vi "ELVIS III v1.0 Configure DMAs.vi"(7 "DMA Type":string, 8 "error in (no error)":errorcluster, 10 "Channel Names":string[](array[string]), 11 "ELVIS III FPGA Ref":T1) -> (0 "error out":errorcluster, 3 "ELVIS III FPGA Ref":T1)   [LabVIEW 2021]
uses:
  <vilib>/myRIO/Common/Instrument Driver Framework/Utilities/typedefs/Generic FPGA Reference.ctl
  <vilib>/myRIO/Common/Instrument Driver Framework/ELVIS III v1.0/Resource Manager/typedefs/ELVIS III IO Config FPGA Reference.ctl
  <vilib>/myRIO/Common/Instrument Driver Framework/myRIO v1.0/Resource Manager/vis/myRIO v1.0 Block Write Configuration.vi
  <vilib>/rvi/interface/common/niFpgaWaitOnOcc.vi
  <vilib>/rvi/interface/nirviMethod/nirviMethod.xnode
  <vilib>/FPGAPlugInAG/Dynamic/niLvFpga_ConfigureFifo_Dynamic.vi
  <vilib>/rvi/errors/niLvFpgaMergeErrorWithErrorCode.vi
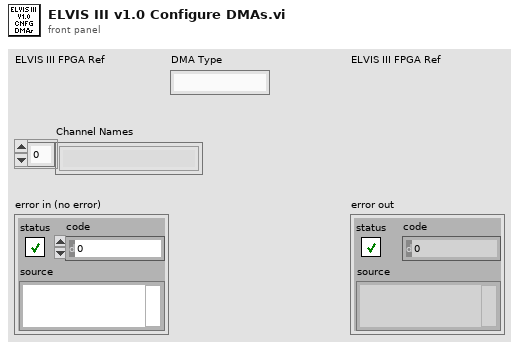
[diagram p1: front panel]
types:
  T1 = typedef "Generic FPGA Reference.ctl" = refnum<k20>
  T2 = typedef "ELVIS III IO Config FPGA Reference.ctl" = refnum<k20>
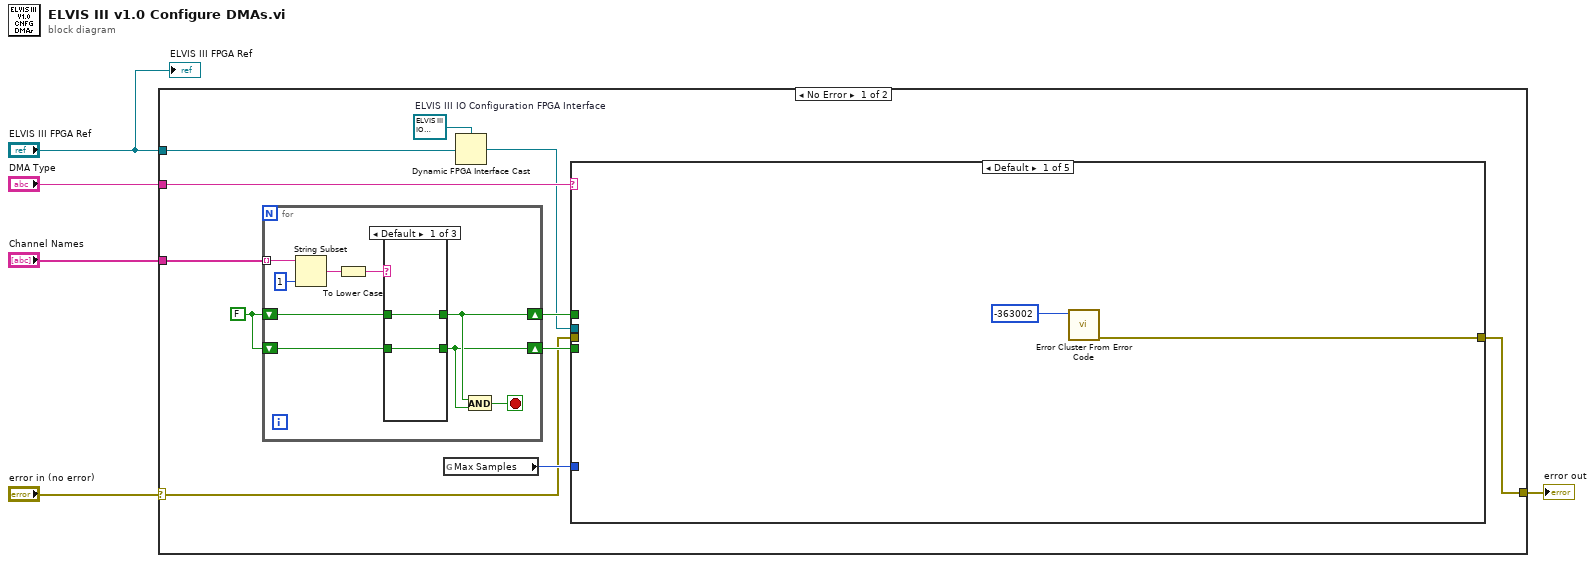
[diagram p0: block diagram]
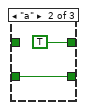
[diagram p2: hidden frame]
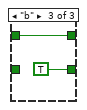
[diagram p3: hidden frame]
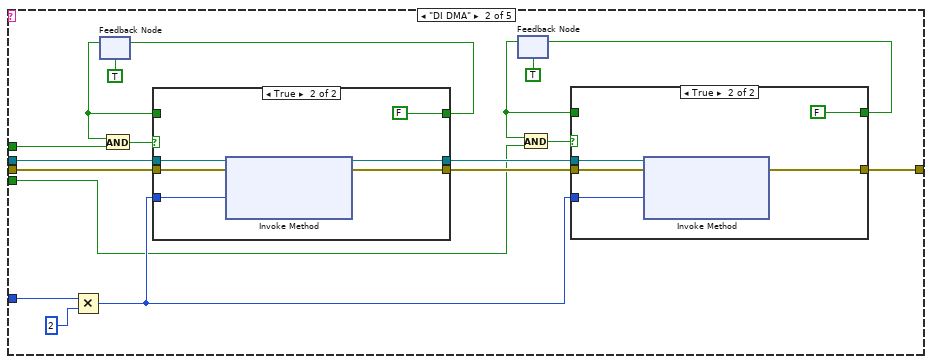
[diagram p4: hidden frame]
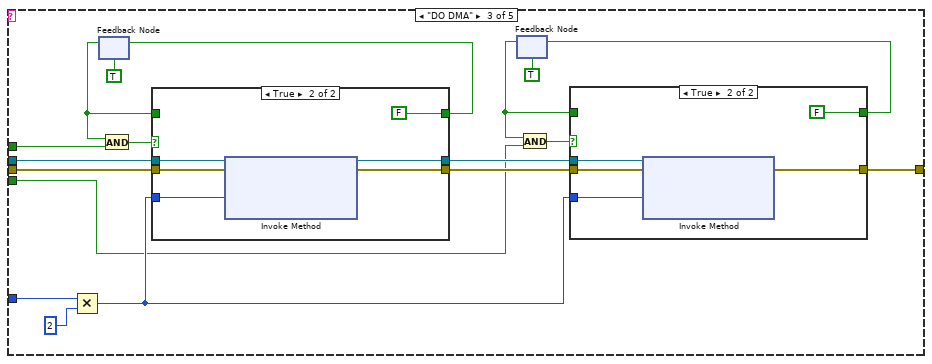
[diagram p7: hidden frame]
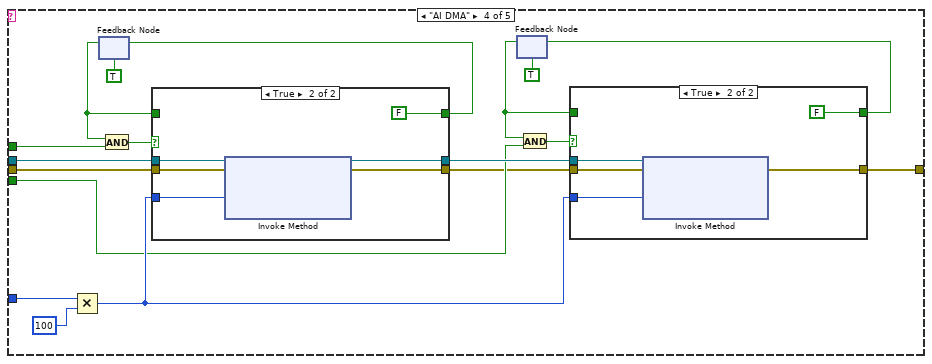
[diagram p10: hidden frame]
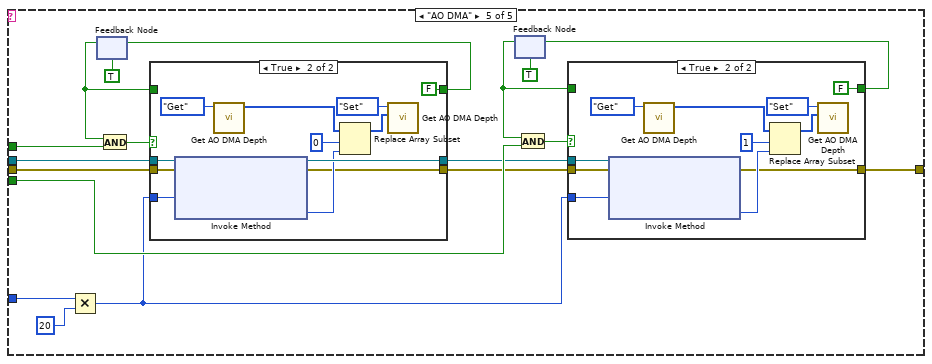
[diagram p13: hidden frame]
diagram:
  n1 = case shown="No Error" "error in (no error)" {
    selector: "error in (no error)" -> [w7 w182]
    tunnel: [w6 w182] -> w4
    tunnel: "ELVIS III FPGA Ref" -> [w16 _]
    tunnel: "DMA Type" -> [w10 _]
    tunnel: "Channel Names" -> [w9 _]
    frame No Error {
      w11 = FALSE
      w15 = T2 refnum  # ELVIS III IO Configuration FPGA Interface
      n2 = for {
        tunnel: w9 -> [w25] mode=indexing
        shift-right: [w19] -> w12
        shift-left: w11 -> [w21]
        shift-right: [w18] -> w13
        shift-left: w11 -> [w20]
        stop <- w17 stop-if-true
        n3 = String Subset(string=w25, length (rest)=1 ("length (rest)")) -> (substring=w23:string)  [unwired: 1 in]
        n4 = To Lower Case(string=w23) -> (all lower case string=w22:string)
        n5 = case shown="Default" w22 {
          tunnel: [w27 TRUE w30] -> w19
          tunnel: w21 -> [w27 _ w30]
          tunnel: [w26 w28 TRUE] -> w18
          tunnel: w20 -> [w26 w28 _]
          frame Default {
          }
          frame "a" {
          }
          frame "b" {
          }
        }
        n6 = And(x=w19, y=w18) -> (x .and. y?=w17:bool)
      }
      n7 = global read "myRIO v1.0 Block Write Configuration.vi" "Max Samples"() -> (w14:u32)
      n8 = Dynamic FPGA Interface Cast(Session In=w15, Type=w16) -> (Session Out=w8:T2)
      n9 = case shown="Default" w10 {
        tunnel: w12 -> [_ w39 w72 w108 w150]
        tunnel: w13 -> [_ w36 w69 w106 w144]
        tunnel: w14 -> [_ w35 w68 w105 w142]
        tunnel: w8 -> [_ w38 w70 w107 w140]
        tunnel: w7 -> [_ w37 w71 w102 w138]
        tunnel: [w32 w34 w73 w104 w136] -> w6
        frame Default {
          n10 = call <vilib>:"Error Cluster From Error Code.vi"("error code (0)"=-363002) -> ("error out"=w32:errorcluster)  [unwired: 8 in]
        }
        frame "DI DMA" {
          n11 = Multiply(x=w35, y=u32 2) -> (x*y=w42:u32)
          n12 = feedback #1(TRUE) -> (w48:bool)
          n13 = And(x=w48, y=w39) -> (x .and. y?=w49:bool)
          n14 = case shown="True" w49 {
            tunnel: [w61 FALSE] -> w50
            tunnel: w48 -> [w61 _]
            tunnel: w42 -> [_ w66]
            tunnel: w38 -> [w60 w65]
            tunnel: [w60 w64] -> w41
            tunnel: [w59 w63] -> w40
            tunnel: w37 -> [w59 w62]
            frame False {
            }
            frame True {
              n15 = xnode "Invoke Method"("FPGA VI Reference In"=w65, "error in"=w62, "Requested Depth"=w66) -> ("FPGA VI Reference Out"=w64:T2, "error out"=w63:errorcluster)  [unwired: 1 out]
            }
          }
          n16 = feedback-in #1(w50) -> ()
          n17 = feedback #2(TRUE) -> (w47:bool)
          n18 = And(x=w47, y=w36) -> (x .and. y?=w46:bool)
          n19 = case shown="True" w46 {
            tunnel: [w53 FALSE] -> w45
            tunnel: w47 -> [w53 _]
            tunnel: w42 -> [_ w57]
            tunnel: w41 -> [_ w56]
            tunnel: [w52 w55] -> w34
            tunnel: w40 -> [w52 w54]
            frame False {
            }
            frame True {
              n20 = xnode "Invoke Method"("FPGA VI Reference In"=w56, "error in"=w54, "Requested Depth"=w57) -> ("error out"=w55:errorcluster)  [unwired: 2 out]
            }
          }
          n21 = feedback-in #2(w45) -> ()
        }
        frame "DO DMA" {
          n22 = Multiply(x=w68, y=u32 2) -> (x*y=w76:u32)
          n23 = feedback #3(TRUE) -> (w82:bool)
          n24 = And(x=w82, y=w72) -> (x .and. y?=w83:bool)
          n25 = case shown="True" w83 {
            tunnel: [w95 FALSE] -> w84
            tunnel: w82 -> [w95 _]
            tunnel: w76 -> [_ w100]
            tunnel: w70 -> [w94 w99]
            tunnel: [w94 w98] -> w75
            tunnel: [w93 w97] -> w74
            tunnel: w71 -> [w93 w96]
            frame False {
            }
            frame True {
              n26 = xnode "Invoke Method"("FPGA VI Reference In"=w99, "error in"=w96, "Requested Depth"=w100) -> ("FPGA VI Reference Out"=w98:T2, "error out"=w97:errorcluster)  [unwired: 1 out]
            }
          }
          n27 = feedback-in #3(w84) -> ()
          n28 = feedback #4(TRUE) -> (w81:bool)
          n29 = And(x=w81, y=w69) -> (x .and. y?=w80:bool)
          n30 = case shown="True" w80 {
            tunnel: [w87 FALSE] -> w79
            tunnel: w81 -> [w87 _]
            tunnel: w76 -> [_ w91]
            tunnel: w75 -> [_ w90]
            tunnel: [w86 w89] -> w73
            tunnel: w74 -> [w86 w88]
            frame False {
            }
            frame True {
              n31 = xnode "Invoke Method"("FPGA VI Reference In"=w90, "error in"=w88, "Requested Depth"=w91) -> ("error out"=w89:errorcluster)  [unwired: 2 out]
            }
          }
          n32 = feedback-in #4(w79) -> ()
        }
        frame "AI DMA" {
          n33 = Multiply(x=w105, y=u32 100) -> (x*y=w110:u32)
          n34 = feedback #5(TRUE) -> (w116:bool)
          n35 = And(x=w116, y=w108) -> (x .and. y?=w117:bool)
          n36 = case shown="True" w117 {
            tunnel: [w129 FALSE] -> w118
            tunnel: w116 -> [w129 _]
            tunnel: w110 -> [_ w134]
            tunnel: w107 -> [w128 w133]
            tunnel: [w128 w132] -> w109
            tunnel: [w127 w131] -> w103
            tunnel: w102 -> [w127 w130]
            frame False {
            }
            frame True {
              n37 = xnode "Invoke Method"("FPGA VI Reference In"=w133, "error in"=w130, "Requested Depth"=w134) -> ("FPGA VI Reference Out"=w132:T2, "error out"=w131:errorcluster)  [unwired: 1 out]
            }
          }
          n38 = feedback-in #5(w118) -> ()
          n39 = feedback #6(TRUE) -> (w115:bool)
          n40 = And(x=w115, y=w106) -> (x .and. y?=w114:bool)
          n41 = case shown="True" w114 {
            tunnel: [w121 FALSE] -> w113
            tunnel: w115 -> [w121 _]
            tunnel: w110 -> [_ w125]
            tunnel: w109 -> [_ w124]
            tunnel: [w120 w123] -> w104
            tunnel: w103 -> [w120 w122]
            frame False {
            }
            frame True {
              n42 = xnode "Invoke Method"("FPGA VI Reference In"=w124, "error in"=w122, "Requested Depth"=w125) -> ("error out"=w123:errorcluster)  [unwired: 2 out]
            }
          }
          n43 = feedback-in #6(w113) -> ()
        }
        frame "AO DMA" {
          n44 = Multiply(x=w142, y=u32 20) -> (x*y=w141:u32)
          n45 = feedback #7(TRUE) -> (w149:bool)
          n46 = And(x=w149, y=w150) -> (x .and. y?=w151:bool)
          n47 = case shown="True" w151 {
            tunnel: [w169 FALSE] -> w152
            tunnel: w149 -> [w169 _]
            tunnel: w141 -> [_ w180]
            tunnel: w140 -> [w168 w179]
            tunnel: [w168 w178] -> w139
            tunnel: w138 -> [w167 w171]
            tunnel: [w167 w170] -> w137
            frame False {
            }
            frame True {
              n48 = xnode "Invoke Method"("FPGA VI Reference In"=w179, "error in"=w171, "Requested Depth"=w180) -> ("FPGA VI Reference Out"=w178:T2, "error out"=w170:errorcluster, "Actual Depth"=w172:u32)
              n49 = call <vilib>:"Get AO DMA Depth.vi"("Action"=enum16{"Get", "Set"}."Get") -> ("DMA Depth Out"=w175:u32[])  [unwired: 9 in, 1 out]
              n50 = Replace Array Subset(array=w175, new element=w172, index=0) -> (w174:u32[])
              n51 = call <vilib>:"Get AO DMA Depth.vi"("DMA Depth In"=w174, "Action"=enum16{"Get", "Set"}."Set") -> ()  [unwired: 8 in, 2 out]
            }
          }
          n52 = feedback-in #7(w152) -> ()
          n53 = feedback #8(TRUE) -> (w148:bool)
          n54 = And(x=w148, y=w144) -> (x .and. y?=w147:bool)
          n55 = case shown="True" w147 {
            tunnel: [w155 FALSE] -> w146
            tunnel: w148 -> [w155 _]
            tunnel: w141 -> [_ w165]
            tunnel: w139 -> [_ w164]
            tunnel: w137 -> [w154 w157]
            tunnel: [w154 w156] -> w136
            frame False {
            }
            frame True {
              n56 = xnode "Invoke Method"("FPGA VI Reference In"=w164, "error in"=w157, "Requested Depth"=w165) -> ("error out"=w156:errorcluster, "Actual Depth"=w158:u32)  [unwired: 1 out]
              n57 = call <vilib>:"Get AO DMA Depth.vi"("Action"=enum16{"Get", "Set"}."Get") -> ("DMA Depth Out"=w161:u32[])  [unwired: 9 in, 1 out]
              n58 = Replace Array Subset(array=w161, new element=w158, index=1) -> (w162:u32[])
              n59 = call <vilib>:"Get AO DMA Depth.vi"("DMA Depth In"=w162, "Action"=enum16{"Get", "Set"}."Set") -> ()  [unwired: 8 in, 2 out]
            }
          }
          n60 = feedback-in #8(w146) -> ()
        }
      }
    }
    frame Error {
    }
  }
  "error out" <- w4
  "ELVIS III FPGA Ref" <- "ELVIS III FPGA Ref"
